vi "Set Comparison String for Config Params Verification.vi"(4 "XPG Serial Number":string) -> (0 "error out":errorcluster, 1 "Comparison String":string)   [LabVIEW 2010]
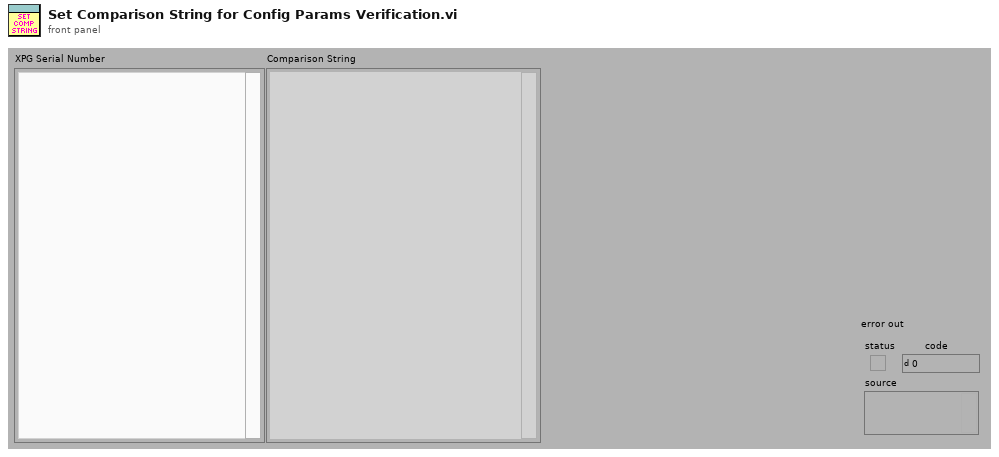
[diagram p1: front panel]
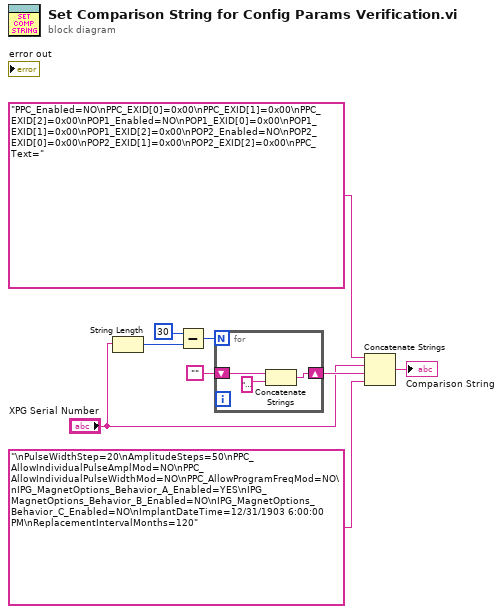
[diagram p0: block diagram]
diagram:
  n1 = String Length(string="XPG Serial Number") -> (length=w9:i32)
  n2 = Subtract(x=30, y=w9) -> (x-y=w7:i32)
  n3 = for {
    N: w7 -> [_]
    shift-right: [w11] -> w5
    shift-left: "" -> [w12]
    n4 = Concatenate Strings(w12, "\u0000" ("String 2")) -> (w11:string)
  }
  n5 = Concatenate Strings("PPC_Enabled=NO\nPPC_EXID[0]=0x00\nPPC_EXID[1]=0x00\nPPC_EXID[2]=0x00\nPOP1_Enabled=NO\nPOP1_EXID[0]=0x00\nPOP1_EXID[1]=0x00\nPOP1_EXID[2]=0x00\nPOP2_Enabled=NO\nPOP2_EXID[0]=0x00\nPOP2_EXID[1]=0x00\nPOP2_EXID[2]=0x00\nPPC_Text=" ("String"), "XPG Serial Number", w5, "\nPulseWidthStep=20\nAmplitudeSteps=50\nPPC_AllowIndividualPulseAmplMod=NO\nPPC_AllowIndividualPulseWidthMod=NO\nPPC_AllowProgramFreqMod=NO\nIPG_MagnetOptions_Behavior_A_Enabled=YES\nIPG_MagnetOptions_Behavior_B_Enabled=NO\nIPG_MagnetOptions_Behavior_C_Enabled=NO\nImplantDateTime=12/31/1903 6:00:00 PM\nReplacementIntervalMonths=120" ("String")) -> (→"Comparison String":string)
